vi "HOST.vi"(8 "Стоп":bool, 9 "Стоп GoTo":bool, 10 "Погнали!":bool, 11 "Куда едем?":T1(ring)) -> (3 "Текущая позиция":dbl)   [LabVIEW 2018]
panel:
  out "IsTriggered":bool
  in  "IsActiveLow":bool
  in  "IsEnabled":bool
  in  "Speed 2":dbl
  in  "Port Name":string="COM1"
  out "Готово":bool
  in  "Тест":bool
  in  "Стоп_тест":bool
  in  "StepMultiplicationFactor":dbl=1.0
  in  "StepDivisor":i32(ring)=8 items=["D1"=1, "D2"=2, "D4"=4, "D8"=8, "D16"=16, "D32"=32]
  in  "Speed":dbl=1000.0
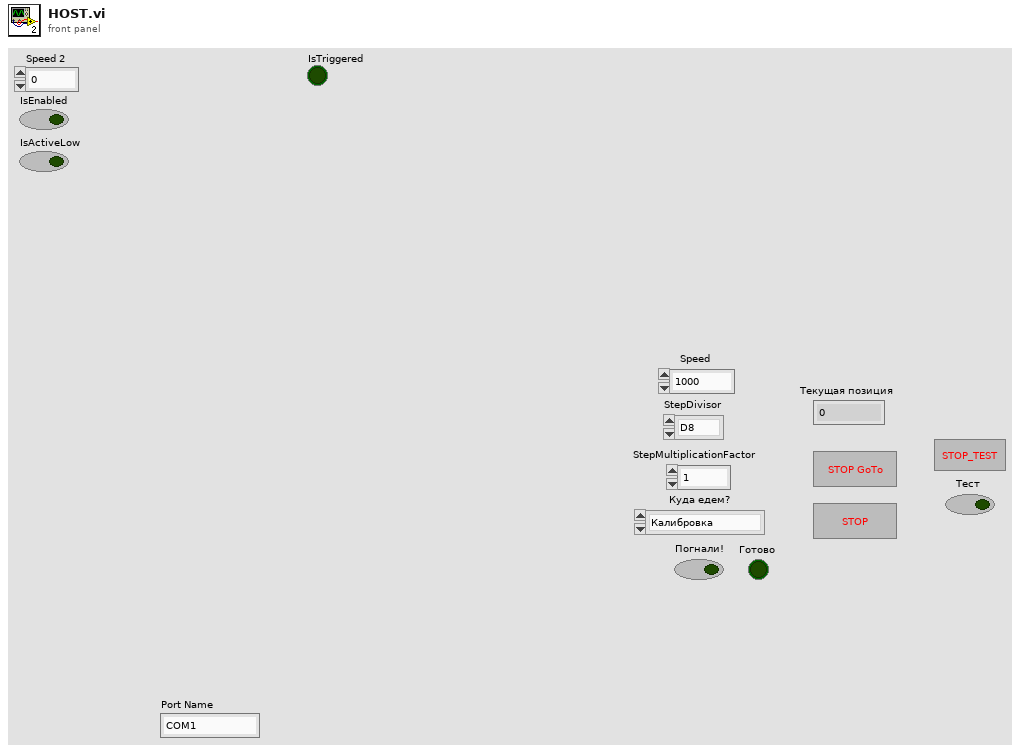
[diagram p1: front panel]
types:
  T1 = enum16{"Калибровка", "Первое стекло", "Второе стекло", "Третье стекло", "Четвертое стекло"}
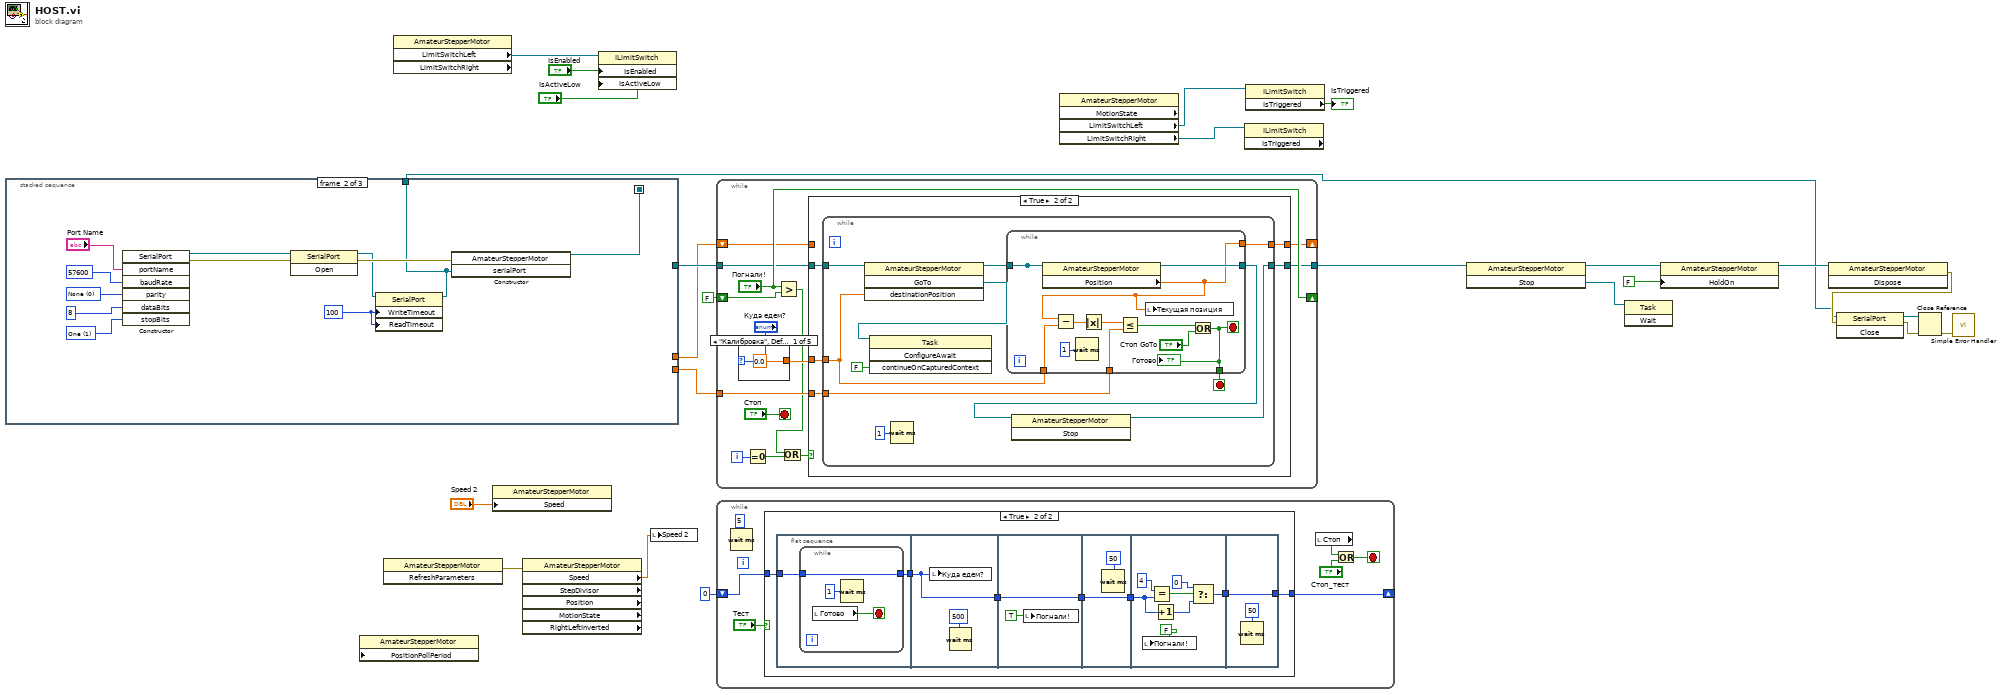
[diagram p0: block diagram]
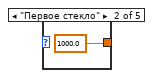
[diagram p3: hidden frame]
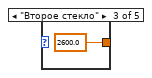
[diagram p4: hidden frame]
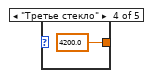
[diagram p5: hidden frame]
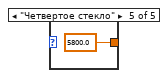
[diagram p6: hidden frame]
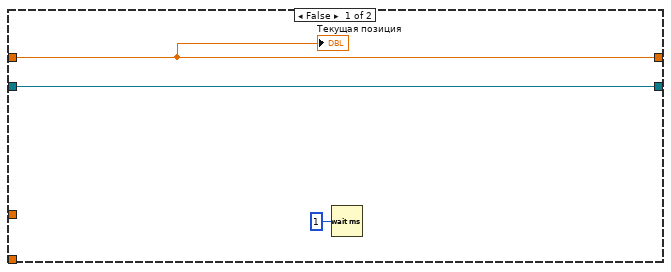
[diagram p7: hidden frame]
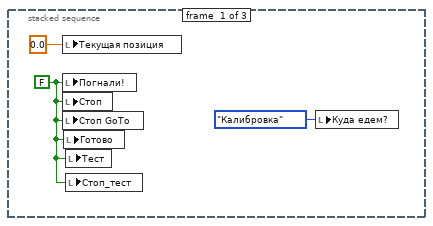
[diagram p8: hidden frame]
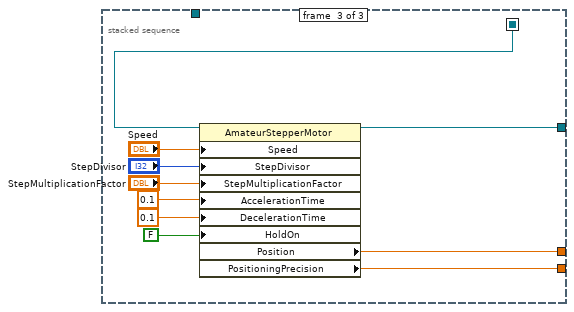
[diagram p9: hidden frame]
diagram:
  n1 = stacked-sequence {
    seq-local: [_ w32 _] -> [_ _ w47]
    tunnel: [_ _ w46] -> w21
    tunnel: [_ _ w42] -> w19
    tunnel: [_ _ w41] -> w18
    tunnel: [_ w29 _] -> w11
    frame #0 {
      w27 = FALSE
      n2 = local write "Текущая позиция"(0.0 ("Текущая позиция")) -> ()
      n3 = local write "Погнали!"(w27) -> ()
      n4 = local write "Стоп"(w27) -> ()
      n5 = local write "Стоп GoTo"(w27) -> ()
      n6 = local write "Готово"(w27) -> ()
      n7 = local write "Тест"(w27) -> ()
      n8 = local write "Стоп_тест"(w27) -> ()
      n9 = local write "Куда едем?"(T1."Калибровка" ("Куда едем?")) -> ()
    }
    frame #1 {
      w30 = 100 ("WriteTimeout")
      w39 = 1 items=["None", "One", "Two", "OnePointFive"] ("stopBits")
      w34 = 0 items=["None", "Odd", "Even", "Mark", "Space"] ("parity")
      n10 = constructor class="SerialPort"("portName"="Port Name", "baudRate"=57600, "parity"=w34, "dataBits"=8, "stopBits"=w39) -> (reference out=w37:refnum<k24>, error out=w36:errorcluster)  [unwired: 3 in, 6 out]
      n11 = invoke class="SerialPort" method="Open"(reference=w37, error in=w36) -> (reference out=w31:refnum<k24>, error out=w40:errorcluster)  [unwired: 1 in, 1 out]
      n12 = property class="SerialPort"(reference=w31, "WriteTimeout"=w30, "ReadTimeout"=w30) -> (reference out=w29:refnum<k24>)  [unwired: 1 in, 1 out]
      n13 = constructor class="AmateurStepperMotor"(error in=w40, "serialPort"=w29) -> (reference out=w32:refnum<k24>)  [unwired: 2 in, 3 out]
    }
    frame #2 {
      n14 = property class="AmateurStepperMotor"(reference=w47, "Speed"="Speed", "StepDivisor"="StepDivisor", "StepMultiplicationFactor"="StepMultiplicationFactor", "AccelerationTime"=0.1, "DecelerationTime"=0.1, "HoldOn"=FALSE) -> (reference out=w46:refnum<k24>, "Position"=w42:dbl, "PositioningPrecision"=w41:dbl)  [unwired: 1 in, 1 out]
    }
  }
  n15 = property class="AmateurStepperMotor" props=["PositionPollPeriod"]() -> ()  [unwired: 3 in, 2 out]
  n16 = invoke class="AmateurStepperMotor" method="RefreshParameters"() -> (error out=w8:errorcluster)  [unwired: 3 in, 2 out]
  n17 = property class="AmateurStepperMotor" props=["LimitSwitchLeft", "LimitSwitchRight"]() -> ("LimitSwitchLeft"=w4:refnum<k24>)  [unwired: 2 in, 3 out]
  n18 = property class="AmateurStepperMotor"("Speed"="Speed 2") -> ()  [unwired: 2 in, 2 out]
  n19 = property class="AmateurStepperMotor" props=["Speed", "StepDivisor", "Position", "MotionState", "RightLeftInverted"](error in=w8) -> ("Speed"=w9:dbl)  [unwired: 1 in, 6 out]
  n20 = property class="ILimitSwitch"(reference=w4, "IsEnabled"="IsEnabled", "IsActiveLow"="IsActiveLow") -> ()  [unwired: 1 in, 2 out]
  n21 = local write "Speed 2"(w9) -> ()
  n22 = while {
    tunnel: w21 -> [w61]
    shift-right: ["Погнали!"] -> _
    shift-left: FALSE ("Поехали!") -> [w63]
    tunnel: [w60] -> w20
    shift-right: [w58] -> _
    shift-left: w19 -> [w59]
    tunnel: w18 -> [w57]
    i -> [w53]
    stop <- "Стоп" stop-if-true
    n23 = case shown="\"Калибровка\", Default" "Куда едем?" {
      tunnel: [0.0 1000.0 2600.0 4200.0 5800.0] -> w55
      frame "Калибровка", Default {
      }
      frame "Первое стекло" {
      }
      frame "Второе стекло" {
      }
      frame "Третье стекло" {
      }
      frame "Четвертое стекло" {
      }
    }
    n24 = Equal To 0?(x=w53) -> (x = 0?=w52:bool)
    n25 = Greater?(x="Погнали!", y=w63) -> (0:w51:bool)
    n26 = Or(x=w51, y=w52) -> (x .or. y?=w54:bool)
    n27 = case shown="True" w54 {
      tunnel: w55 -> [_ w77]
      tunnel: w61 -> [w71 w76]
      tunnel: [w71 w75] -> w60
      tunnel: w59 -> [w70 _]
      tunnel: [w70 w74] -> w58
      tunnel: w57 -> [_ w73]
      frame False {
        n28 = Wait (ms)(milliseconds to wait=u32 1) -> ()  [unwired: 1 out]
        "Текущая позиция" <- w70
      }
      frame True {
        n29 = while {
          tunnel: w77 -> [w83]
          tunnel: w76 -> [w86]
          tunnel: [w80] -> w75
          tunnel: [w85] -> w74
          tunnel: w73 -> [w82]
          stop <- w84 stop-if-true
          n30 = invoke class="AmateurStepperMotor" method="GoTo"(reference=w86, "destinationPosition"=w83) -> (reference out=w88:refnum<k24>, "GoTo"=w89:refnum<k24>)  [unwired: 2 in, 2 out]
          n31 = invoke class="Task" method="ConfigureAwait"(reference=w89, "continueOnCapturedContext"=FALSE) -> ()  [unwired: 2 in, 4 out]
          n32 = Wait (ms)(milliseconds to wait=u32 1) -> ()  [unwired: 1 out]
          n33 = while {
            tunnel: [w93] -> w85
            tunnel: w88 -> [w90]
            tunnel: [w100] -> w81
            tunnel: [w92] -> w84
            tunnel: w83 -> [w98]
            tunnel: w82 -> [w96]
            tunnel: [w90] -> w78
            stop <- w92 stop-if-true
            n34 = property class="AmateurStepperMotor"(reference=w90) -> (reference out=w100:refnum<k24>, "Position"=w93:dbl)  [unwired: 1 in, 1 out]
            n35 = Subtract(x=w93, y=w98) -> (x-y=w99:dbl)
            n36 = Wait (ms)(milliseconds to wait=u32 1) -> ()  [unwired: 1 out]
            n37 = Absolute Value(x=w99) -> (abs(x)=w97:dbl)
            n38 = Less Or Equal?(x=w97, y=w96) -> (x <= y?=w95:bool)
            n39 = local write "Текущая позиция"(w93) -> ()
            n40 = Or(x=w95, y="Стоп GoTo") -> (x .or. y?=w92:bool)
            "Готово" <- w92
          }
          n41 = invoke class="AmateurStepperMotor" method="Stop"(reference=w81) -> (reference out=w80:refnum<k24>)  [unwired: 2 in, 2 out]
        }
      }
    }
  }
  n42 = while {
    shift-right: [w101] -> _
    shift-left: 0 -> [w102]
    stop <- w105 stop-if-true
    n43 = Wait (ms)(milliseconds to wait=u32 5) -> ()  [unwired: 1 out]
    n44 = case shown="True" "Тест" {
      tunnel: w102 -> [w108 w115]
      tunnel: [w108 w112] -> w101
      frame False {
      }
      frame True {
        n45 = flat-sequence {
          tunnel: w115 -> [w117]
          tunnel: [w116] -> w110
          tunnel: [w122] -> w111
          tunnel: w110 -> [w122]
          tunnel: [w124] -> w113
          tunnel: w111 -> [w124]
          tunnel: [w125] -> w114
          tunnel: w113 -> [w125]
          tunnel: w114 -> [w130]
          tunnel: [w128] -> w109
          tunnel: [w135] -> w112
          tunnel: w109 -> [w135]
          frame #0 {
            n46 = while {
              tunnel: w117 -> [w120]
              tunnel: [w120] -> w116
              stop <- w119 stop-if-true
              n47 = local read "Готово"() -> (w119:bool)
              n48 = Wait (ms)(milliseconds to wait=u32 1) -> ()  [unwired: 1 out]
            }
          }
          frame #1 {
            n49 = local write "Куда едем?"(w122) -> ()
            n50 = Wait (ms)(milliseconds to wait=u32 500) -> ()  [unwired: 1 out]
          }
          frame #2 {
            n51 = local write "Погнали!"(TRUE ("Погнали!")) -> ()
          }
          frame #3 {
            n52 = Wait (ms)(milliseconds to wait=u32 50) -> ()  [unwired: 1 out]
          }
          frame #4 {
            n53 = local write "Погнали!"(FALSE ("Погнали!")) -> ()
            n54 = Equal?(x=4, y=w130) -> (x = y?=w132:bool)
            n55 = Increment(x=w130) -> (x+1=w129:i32)
            n56 = Select(t=0, s=w132, f=w129) -> (s? t:f=w128:i32)
          }
          frame #5 {
            n57 = Wait (ms)(milliseconds to wait=u32 50) -> ()  [unwired: 1 out]
          }
        }
      }
    }
    n58 = local read "Стоп"() -> (w104:bool)
    n59 = Or(x=w104, y="Стоп_тест") -> (x .or. y?=w105:bool)
  }
  n60 = property class="AmateurStepperMotor" props=["MotionState", "LimitSwitchLeft", "LimitSwitchRight"]() -> (reference=w7:refnum<k24>, "LimitSwitchLeft"=w6:refnum<k24>, "LimitSwitchRight"=w5:refnum<k24>)  [unwired: 1 in, 3 out]
  n61 = property class="ILimitSwitch" props=["IsTriggered"](reference=w5) -> ()  [unwired: 1 in, 3 out]
  n62 = property class="ILimitSwitch"(reference=w6) -> ("IsTriggered"=→"IsTriggered":bool)  [unwired: 1 in, 2 out]
  n63 = invoke class="AmateurStepperMotor" method="Stop"(reference=w20) -> (reference out=w24:refnum<k24>, "Stop"=w25:refnum<k24>)  [unwired: 2 in, 1 out]
  n64 = invoke class="Task" method="Wait"(reference=w25) -> ()  [unwired: 2 in, 3 out]
  n65 = property class="AmateurStepperMotor"(reference=w24, "HoldOn"=FALSE) -> (reference out=w23:refnum<k24>)  [unwired: 1 in, 1 out]
  n66 = invoke class="AmateurStepperMotor" method="Dispose"(reference=w23) -> (error out=w12:errorcluster)  [unwired: 2 in, 2 out]
  n67 = invoke class="SerialPort" method="Close"(reference=w11, error in=w12) -> (reference out=w13:refnum<k24>, error out=w14:errorcluster)  [unwired: 1 in, 1 out]
  n68 = Close Reference(reference=w13, error in (no error)=w14) -> (error out=w15:errorcluster)
  n69 = call <vilib>:"Simple Error Handler.vi"("error in (no error)"=w15) -> ()  [unwired: 1 in, 8 out]
